vi "Test Reference Phase.vi"(8 "error in (no error)":errorcluster, 11 "SR7270 Drivers in":refnum<class "SR7270 Drivers.lvclass">) -> (0 "error out":errorcluster, 3 "SR7270 Drivers out":refnum<class "SR7270 Drivers.lvclass">)   [LabVIEW 2016, in "SR7270 Drivers.lvlib"]
uses:
  SR7270 Drivers.lvlib
  <vilib>/addons/_JKI Toolkits/Caraya/classes/Test/Test.lvclass
  <userlib>/_OpenG.lib/numeric/numeric.llb/Random Number Within Range - DBL__ogtk.vi
  Typedefs/REFMODE--enum.ctl
  Typedefs/VRLOCK--enum.ctl
  <vilib>/addons/_JKI Toolkits/Caraya/classes/Assert/Assert.lvclass
  SR7270 Drivers.lvclass
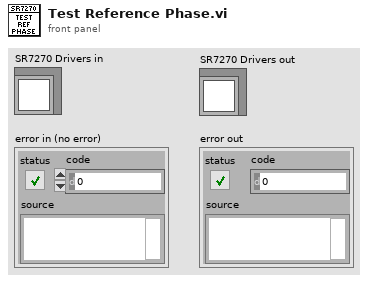
[diagram p1: front panel]
types:
  T1 = typedef "SR7270 Drivers.lvlib/VRLOCK--enum.ctl" = enum16{"Disabled", "Enabled"}
  T2 = typedef "SR7270 Drivers.lvlib/REFMODE--enum.ctl" = enum16{"Single Reference/Virtual Reference", "Dual Harmonic", "Dual Reference"}
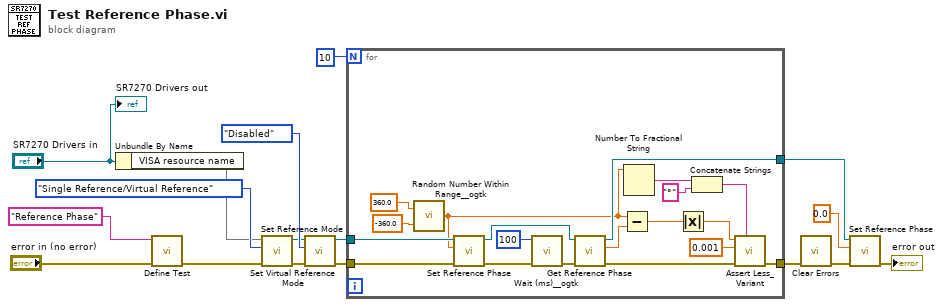
[diagram p0: block diagram]
diagram:
  n1 = Unbundle By Name("SR7270 Drivers in") -> ("VISA resource name"=w2)
  n2 = call <vilib>:"Define Test.vi"("error in (no error)"="error in (no error)", "Label (VI Title)"="Reference Phase") -> ("error out"=w5:errorcluster)  [unwired: 9 in]
  n3 = call "Set Reference Mode.vi"("error in (no error)"=w5, "Reference Mode"=REFMODE--enum."Single Reference/Virtual Reference", "VISA resource name"=w2) -> ("error out"=w8:errorcluster, "VISA resource name out"=w6:refnum<visa-resource-name>)  [unwired: 7 in]
  n4 = call "Set Virtual Reference Mode.vi"("error in (no error)"=w8, "Virtual Reference Lock"=VRLOCK--enum."Disabled", "VISA resource name"=w6) -> ("error out"=w4:errorcluster, "VISA resource name out"=w3:refnum<visa-resource-name>)  [unwired: 7 in]
  n5 = for {
    N: 10 -> [_]
    tunnel: w3 -> [w35]
    tunnel: w4 -> [w30]
    tunnel: [w24] -> w17
    tunnel: [w34] -> w14
    n6 = call-poly <userlib>:"Random Number Within Range__ogtk.vi"("High"=360.0, "Low"=-360.0) -> ("Random Number"=w22:dbl)  [unwired: 3 in]
    n7 = call "Set Reference Phase.vi"("error in (no error)"=w30, "Phase (°)"=w22, "VISA resource name"=w35) -> ("error out"=w31:errorcluster, "VISA resource name out"=w36:refnum<visa-resource-name>)  [unwired: 7 in]
    n8 = call <userlib>:"Wait (ms)__ogtk.vi"("error in (no error)"=w31, "milliseconds to wait"=u32 100) -> ("error out"=w33:errorcluster)  [unwired: 8 in, 1 out]
    n9 = call "Get Reference Phase.vi"("error in (no error)"=w33, "VISA resource name"=w36) -> ("error out"=w25:errorcluster, "Phase (°)"=w21:dbl, "VISA resource name out"=w34:refnum<visa-resource-name>)  [unwired: 7 in]
    n10 = Subtract(x=w22, y=w21) -> (x-y=w20:dbl)
    n11 = Number To Fractional String(number=w22) -> (F-format string=w27:string)  [unwired: 3 in]
    n12 = Absolute Value(x=w20) -> (abs(x)=w19:dbl)
    n13 = Concatenate Strings(w27, "°" ("string")) -> (w23:string)
    n14 = call <vilib>:"Assert Less_Variant.vi"("Label"=w23, "error in (no error)"=w25, "Y"=0.001 ("Phase (°)"), "X"=w19) -> ("error out"=w24:errorcluster)  [unwired: 7 in]
  }
  n15 = call <vilib>:"Clear Errors.vi"("error in (no error)"=w17) -> ("error out"=w12:errorcluster)  [unwired: 5 in, 1 out]
  n16 = call "Set Reference Phase.vi"("error in (no error)"=w12, "Phase (°)"=0.0, "VISA resource name"=w14) -> ("error out"=→"error out":errorcluster)  [unwired: 7 in, 1 out]
  "SR7270 Drivers out" <- "SR7270 Drivers in"
